vi "RP trx test.vi"() -> ()   [LabVIEW 2016]
uses:
  Receiver format.ctl
  RP Transceiver.lvclass
  C:/github/NHMFL_Core/Libraries/Red Pitaya/RP Core/RP Instrument/RP Instrument.lvclass
  RP Instrument/RP Instrument.lvclass/RP Instrument.ctl
  RP Transceiver.lvclass/RP Transceiver.ctl
  RP Instrument/Write Status check delay.vi
  Write Receiver format.vi
  RP Instrument/Write DDS delay.vi
  <vilib>/Utility/file.llb/Write Delimited Spreadsheet (DBL).vi
panel:
  in  "DDS delay":u32=47
  in  "Save":bool
  in  "Sweep F":bool=TRUE
  out "Waveform Graph 2":i16[](graph)
  in  "Number WFRM points":i32=1000000 format="%.0p"
  in  "Flush FIFO":bool
  out "write size":i32
  in  "Receiver format":T1=enum."F-X-Y"
  out "Old data":i32[](array[numeric])
  out "Waveform Graph":dbl[](graph)
  in  "Reset":bool=TRUE
  in  "read size":i32=300
  out "Data out":cdb[](array[numeric])
  out "XY Graph":T2(graph)
  in  "Step":dbl=50000.0 format="%#_6p"
  in  "End":dbl=18000000.0 format="%#_6p"
  in  "Start":dbl=50000.0 format="%#_6p"
  in  "Averaging time":dbl=0.0084
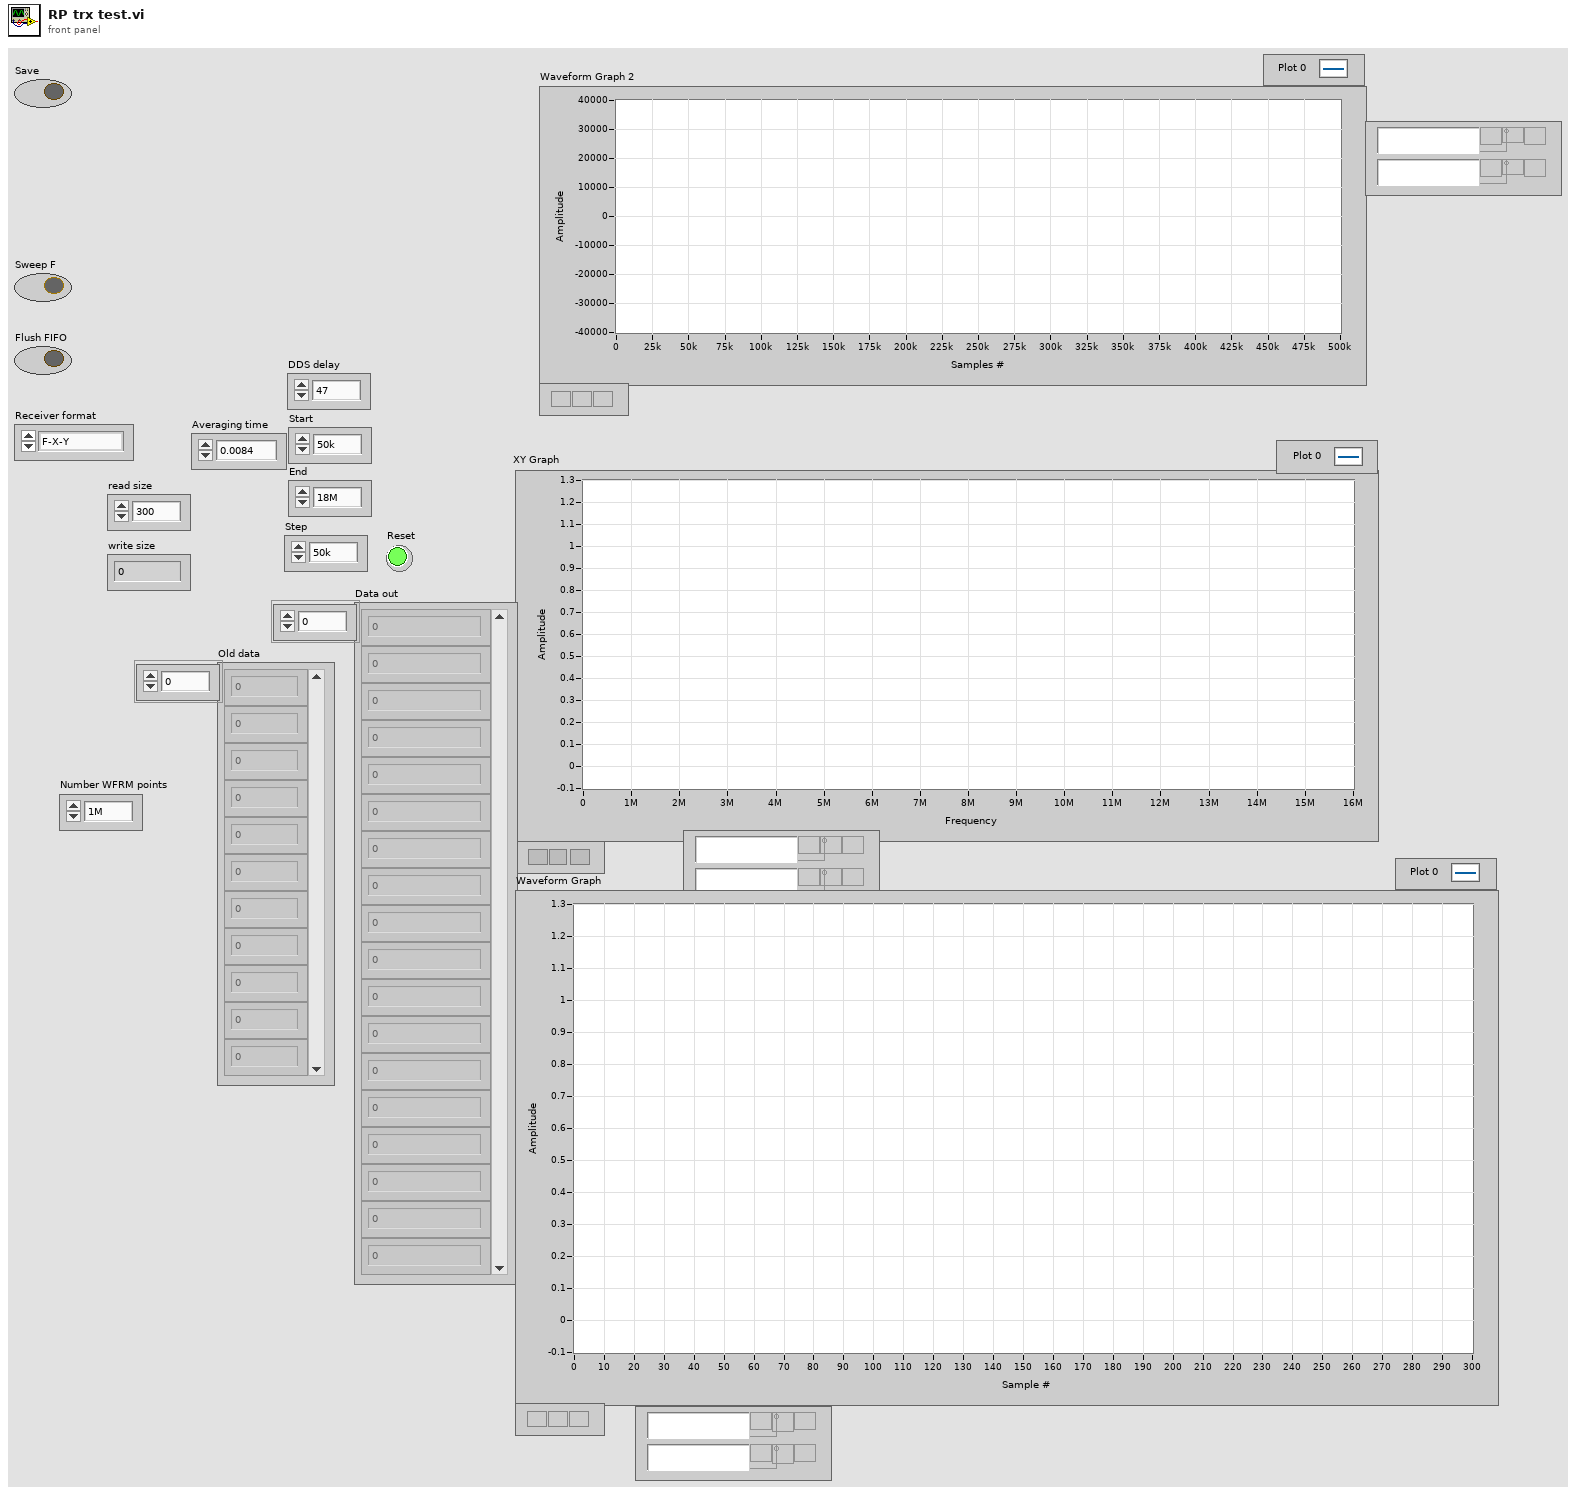
[diagram p1: front panel]
types:
  T1 = typedef "Receiver format.ctl" = enum16{"X-Y-F", "F-X-Y", "X-Y", "X"}
  T2 = cluster{"Frequency out":dbl[], "Volatge out":dbl[]}[]
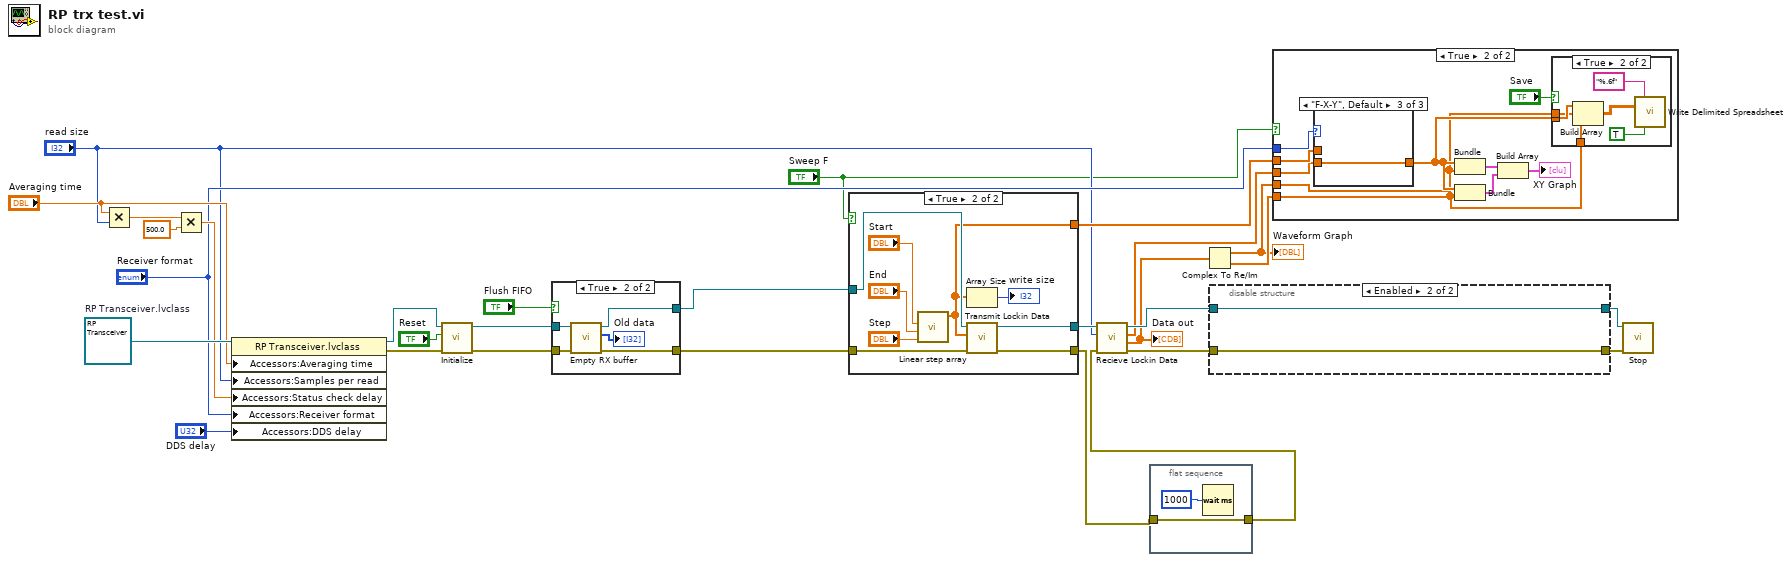
[diagram p0: block diagram]
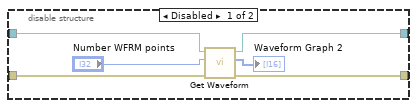
[diagram p2: hidden frame]
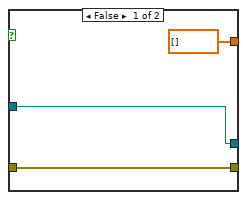
[diagram p7: hidden frame]
diagram:
  w29 = refnum<class "RP Transceiver.lvclass"> refnum  # RP Transceiver.lvclass
  n1 = Multiply(x="Averaging time", y="read size") -> (x*y=w27:dbl)
  n2 = Multiply(x=w27, y=500.0) -> (x*y=w25:dbl)
  n3 = property class="RP Transceiver.lvclass"(reference=w29, "Accessors:Averaging time"="Averaging time", "Accessors:Samples per read"="read size", "Accessors:Status check delay"=w25, "Accessors:Receiver format"="Receiver format", "Accessors:DDS delay"="DDS delay") -> (reference out=w24:refnum<class "RP Transceiver.lvclass">, error out=w23:errorcluster)  [unwired: 1 in]
  n4 = call-dynamic "Initialize.vi"("error in (no error)"=w23, "Reset"="Reset", "RP Transceiver in"=w24) -> ("error out"=w18:errorcluster, "RP Transceiver out"=w19:refnum<class "RP Transceiver.lvclass">)  [unwired: 7 in]
  n5 = case shown="True" "Flush FIFO" {
    tunnel: w19 -> [w31 w36]
    tunnel: w18 -> [w30 w35]
    tunnel: [w31 w34] -> w17
    tunnel: [w30 w33] -> w4
    frame False {
    }
    frame True {
      n6 = call-dynamic "Empty RX buffer.vi"("error in (no error)"=w35, "RP Instrument in"=w36) -> ("error out"=w33:errorcluster, "Data out"=→"Old data":i32[], "RP Instrument out"=w34:refnum<class "RP Transceiver.lvclass">)  [unwired: 7 in]
    }
  }
  n7 = case shown="True" "Sweep F" {
    tunnel: [w37 w45] -> w22
    tunnel: w17 -> [w37 w44]
    tunnel: w4 -> [w38 w43]
    tunnel: [dbl[] [] ("Steps") w42] -> w15
    tunnel: [w38 w40] -> w3
    frame False {
    }
    frame True {
      n8 = call "Linear step array.vi"("Step"="Step", "End"="End", "Start"="Start") -> ("Steps"=w42:dbl[])  [unwired: 8 in]
      n9 = Array Size(array=w42) -> (size(s)=→"write size":i32)
      n10 = call-dynamic "Transmit Lockin Data.vi"("error in (no error)"=w43, "Data"=w42, "RP Transceiver in"=w44) -> ("error out"=w40:errorcluster, "RP Transceiver out"=w45:refnum<class "RP Transceiver.lvclass">)  [unwired: 6 in, 1 out]
    }
  }
  n11 = call-dynamic "Recieve Lockin Data.vi"("error in (no error)"=w2, "Points to read"="read size", "RP Lockin in"=w22) -> ("error out"=w7:errorcluster, "Volatge out"=w13:cdb[], "Frequency out"=w14:dbl[], "RP Lockin out"=w21:refnum<class "RP Transceiver.lvclass">)  [unwired: 5 in]
  "Data out" <- w13
  n12 = flat-sequence {
    tunnel: w3 -> [w50]
    tunnel: [w50] -> w2
    frame #0 {
      n13 = Wait (ms)(milliseconds to wait=u32 1000) -> ()  [unwired: 1 out]
    }
  }
  n14 = Complex To Re/Im(x + iy=w13) -> (x=w9:dbl[], y=w12:dbl[])
  "Waveform Graph" <- w9
  n15 = disable-structure shown="Enabled" {
    disable-tunnel: w21 -> [w56 w57]
    disable-tunnel: [w55 w57] -> w8
    disable-tunnel: w7 -> [w52 w58]
    disable-tunnel: [w51 w58] -> w6
    frame Disabled {
      n16 = call-dynamic "Get Waveform.vi"("error in (no error)"=w52, "Pre-trigger points"="Number WFRM points", "RP Instrument in"=w56) -> ("error out"=w51:errorcluster, "Data out"=→"Waveform Graph 2":i16[], "RP Instrument out"=w55:refnum<class "RP Transceiver.lvclass">)  [unwired: 6 in]
    }
    frame Enabled {
    }
  }
  n17 = case shown="True" "Sweep F" {
    tunnel: "Receiver format" -> [_ w67]
    tunnel: w15 -> [_ w66]
    tunnel: w14 -> [_ w65]
    tunnel: w12 -> [_ w59]
    tunnel: w9 -> [_ w60]
    frame False {
    }
    frame True {
      n18 = case shown="\"F-X-Y\", Default" w67 {
        tunnel: [w75 w76 w77] -> w61
        tunnel: w66 -> [w75 w76 _]
        tunnel: w65 -> [_ _ w77]
        frame "X-Y" {
        }
        frame "X" {
        }
        frame "F-X-Y", Default {
        }
      }
      n19 = Bundle("Frequency out"=w61, w60) -> (w68:cluster{"Frequency out":dbl[], dbl[]})  [unwired: 1 in]
      n20 = Bundle("Frequency out"=w61, w59) -> (w63:cluster{"Frequency out":dbl[], dbl[]})  [unwired: 1 in]
      n21 = Build Array(w68, w63) -> (→"XY Graph":cluster{"Frequency out":dbl[], dbl[]}[])
      n22 = case shown="True" "Save" {
        tunnel: w61 -> [_ w74]
        tunnel: w60 -> [_ w73]
        tunnel: w59 -> [_ w72]
        frame False {
        }
        frame True {
          n23 = Build Array(w74, w73, w72) -> (w71:dbl[][])
          n24 = call-poly <vilib>:"Write Delimited Spreadsheet.vi"("format (%.3f)"="%.6f", "2D data"=w71, "transpose? (no:F)"=TRUE ("transpose? (F)")) -> ()  [unwired: 11 in, 2 out]
        }
      }
    }
  }
  n25 = call-dynamic "Stop.vi"("error in (no error)"=w6, "RP Instrument in"=w8) -> ()  [unwired: 8 in, 2 out]
